vi "case_statement.vi"() -> ()   [LabVIEW 2017]
panel:
  in  "String":string
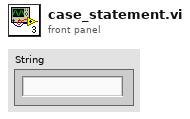
[diagram p1: front panel]
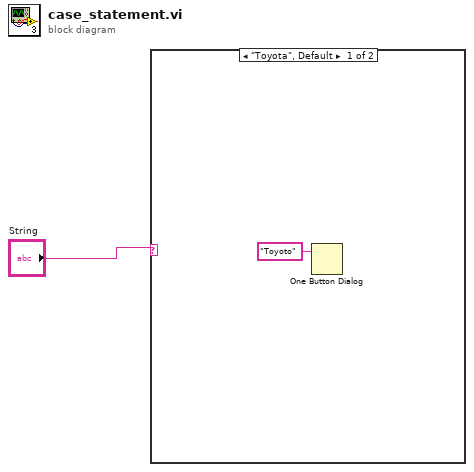
[diagram p0: block diagram]
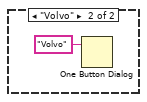
[diagram p2: hidden frame]
diagram:
  n1 = case shown="\"Toyota\", Default" "String" {
    frame "Toyota", Default {
      n2 = One Button Dialog(message="Toyoto") -> ()  [unwired: 1 in, 1 out]
    }
    frame "Volvo" {
      n3 = One Button Dialog(message="Volvo") -> ()  [unwired: 1 in, 1 out]
    }
  }
